vi "Motor_Control.vi"() -> ()   [LabVIEW 2024]
panel:
  out "MotorPosition":i32
  in  "B1":bool
  in  "B10000":bool
  in  "B50000":bool
  in  "B200000":bool
  in  "F200000":bool
  in  "F50000":bool
  in  "F10000":bool
  in  "F1":bool
  in  "Stop":bool
  out "ZMotorTrace":dbl(graph)
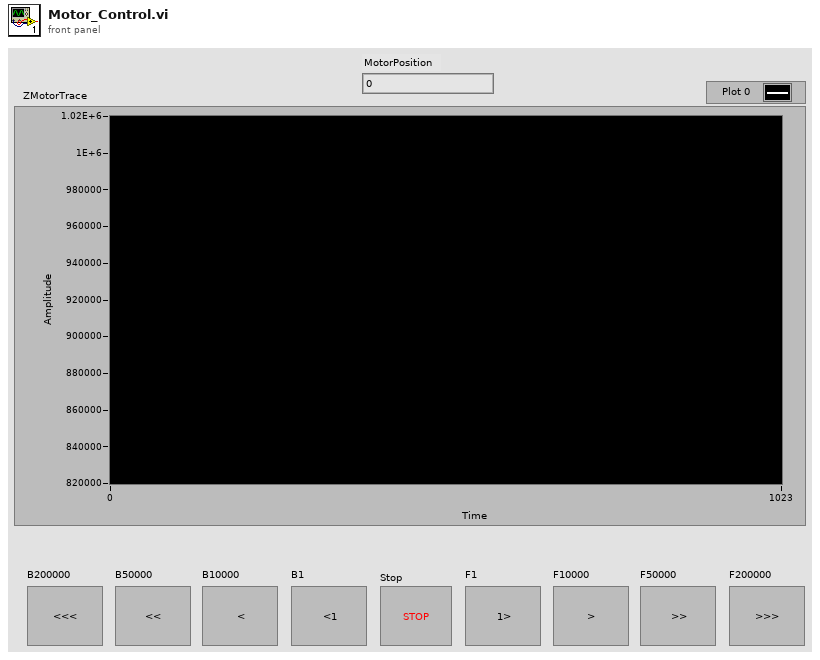
[diagram p1: front panel]
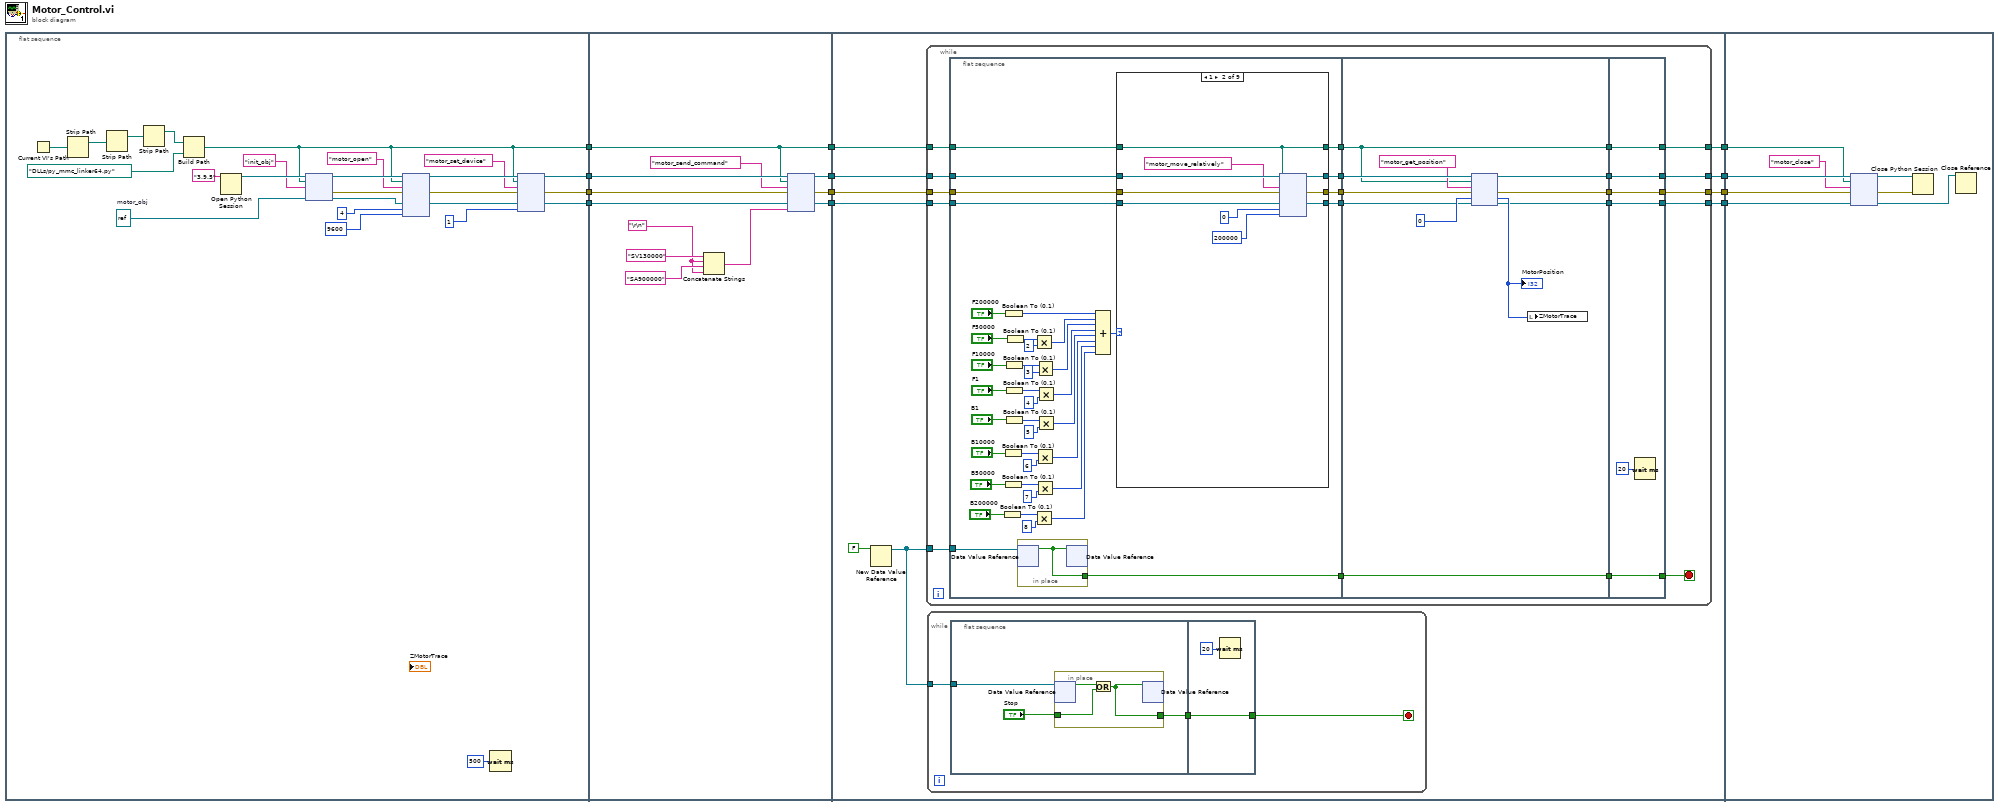
[diagram p0: block diagram]
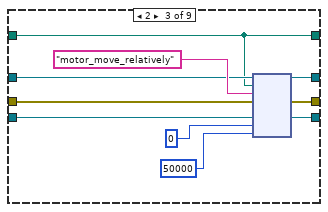
[diagram p3: hidden frame]
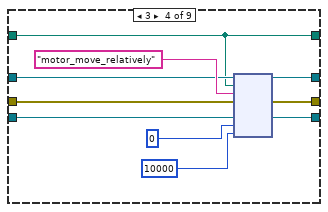
[diagram p4: hidden frame]
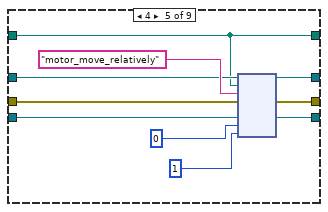
[diagram p5: hidden frame]
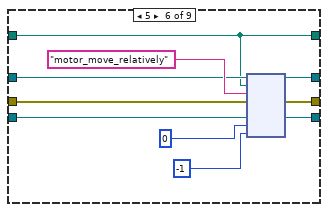
[diagram p6: hidden frame]
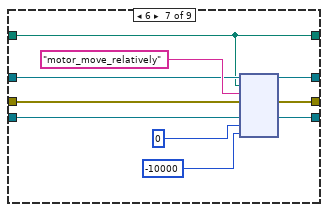
[diagram p7: hidden frame]
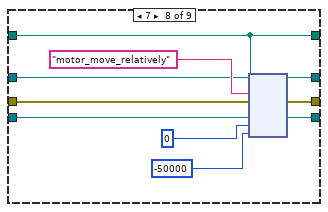
[diagram p8: hidden frame]
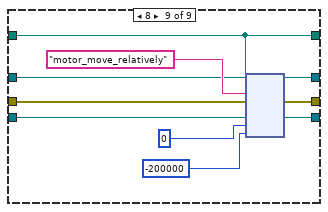
[diagram p9: hidden frame]
diagram:
  n1 = flat-sequence {
    tunnel: [w13] -> w12
    tunnel: [w19] -> w11
    tunnel: [w18] -> w10
    tunnel: [w17] -> w9
    tunnel: w12 -> [w42]
    tunnel: w11 -> [w47]
    tunnel: w10 -> [w46]
    tunnel: w9 -> [w45]
    tunnel: [w42] -> w8
    tunnel: [w41] -> w7
    tunnel: [w40] -> w6
    tunnel: [w39] -> w5
    tunnel: w8 -> [w57]
    tunnel: w7 -> [w56]
    tunnel: w6 -> [w55]
    tunnel: w5 -> [w54]
    tunnel: [w53] -> w4
    tunnel: [w52] -> w3
    tunnel: [w51] -> w2
    tunnel: [w50] -> w1
    tunnel: w4 -> [w238]
    tunnel: w3 -> [w241]
    tunnel: w2 -> [w239]
    tunnel: w1 -> [w240]
    frame #0 {
      w30 = refnum<k38> refnum  # motor_obj
      n2 = Current VI's Path() -> (path=w34:path)
      n3 = Strip Path(path=w34) -> (stripped path=w33:path)  [unwired: 1 out]
      n4 = Strip Path(path=w33) -> (stripped path=w15:path)  [unwired: 1 out]
      n5 = Strip Path(path=w15) -> (stripped path=w14:path)  [unwired: 1 out]
      n6 = Build Path(base path=w14, name or relative path=path "DLLs/py_mmc_linker64.py") -> (appended path=w13:path)
      n7 = Open Python Session(python version="3.9.5" ("Python version")) -> (session out=w35:refnum<k35>)  [unwired: 2 in, 1 out]
      n8 = node(w35, w13, "init_obj" ("function name"), w30) -> (w29:refnum<k35>, w28:errorcluster, w26:refnum<k38>)  [unwired: 1 in, 2 out]
      n9 = node(w29, w13, "motor_open" ("function name"), w28, w26, u8 4 ("COM port select"), 9600 ("COM port select")) -> (w23:refnum<k35>, w22:errorcluster, w21:refnum<k38>)  [unwired: 4 in, 2 out]
      n10 = Wait (ms)(milliseconds to wait=u32 500) -> ()  [unwired: 1 out]
      n11 = node(w23, w13, "motor_set_device" ("function name"), w22, w21, u8 1 ("COM port select")) -> (w19:refnum<k35>, w18:errorcluster, w17:refnum<k38>)  [unwired: 3 in, 2 out]
    }
    frame #1 {
      w38 = "\r\n"
      n12 = Concatenate Strings("SV130000", w38, "SA900000", w38) -> (w44:string)
      n13 = node(w47, w42, "motor_send_command" ("function name"), w46, w45, w44) -> (w41:refnum<k35>, w40:errorcluster, w39:refnum<k38>)  [unwired: 3 in, 2 out]
    }
    frame #2 {
      n14 = New Data Value Reference(data value=FALSE) -> (data value reference=w58:refnum<data-value>)  [unwired: 1 in, 1 out]
      n15 = while {
        tunnel: w58 -> [w90]
        tunnel: w57 -> [w86]
        tunnel: w56 -> [w85]
        tunnel: w55 -> [w84]
        tunnel: w54 -> [w83]
        tunnel: [w77] -> w53
        tunnel: [w75] -> w52
        tunnel: [w73] -> w51
        tunnel: [w71] -> w50
        stop <- w89 stop-if-true
        n16 = flat-sequence {
          tunnel: w90 -> [w131]
          tunnel: [w130] -> w88
          tunnel: w86 -> [w98]
          tunnel: w85 -> [w97]
          tunnel: w84 -> [w96]
          tunnel: w83 -> [w95]
          tunnel: [w94] -> w82
          tunnel: [w93] -> w81
          tunnel: [w92] -> w80
          tunnel: [w91] -> w79
          tunnel: w88 -> [w227]
          tunnel: [w227] -> w87
          tunnel: w82 -> [w226]
          tunnel: w81 -> [w225]
          tunnel: w80 -> [w219]
          tunnel: w79 -> [w221]
          tunnel: [w221] -> w78
          tunnel: [w220] -> w76
          tunnel: [w218] -> w74
          tunnel: [w217] -> w72
          tunnel: [w233] -> w89
          tunnel: w87 -> [w233]
          tunnel: w78 -> [w231]
          tunnel: [w231] -> w77
          tunnel: w76 -> [w230]
          tunnel: [w230] -> w75
          tunnel: [w229] -> w73
          tunnel: w74 -> [w229]
          tunnel: w72 -> [w228]
          tunnel: [w228] -> w71
          frame #0 {
            n17 = Boolean To (0,1)(Boolean="B200000") -> (0, 1=w102:i16)
            n18 = Boolean To (0,1)(Boolean="B10000") -> (0, 1=w110:i16)
            n19 = Boolean To (0,1)(Boolean="B50000") -> (0, 1=w105:i16)
            n20 = Boolean To (0,1)(Boolean="F200000") -> (0, 1=w128:i16)
            n21 = Boolean To (0,1)(Boolean="F10000") -> (0, 1=w121:i16)
            n22 = Boolean To (0,1)(Boolean="F1") -> (0, 1=w117:i16)
            n23 = Boolean To (0,1)(Boolean="B1") -> (0, 1=w113:i16)
            n24 = Boolean To (0,1)(Boolean="F50000") -> (0, 1=w125:i16)
            n25 = in-place {
              in-place-border: [w216] -> w130
              n26 = in-place-dvr #1(w131) -> (w216:bool)  [unwired: 1 out]
              n27 = in-place-dvr #1(w216) -> ()  [unwired: 2 out]
            }
            n28 = Multiply(x=w125, y=i16 2) -> (x*y=w123:i16)
            n29 = Multiply(x=w102, y=i16 8) -> (x*y=w99:i16)
            n30 = Multiply(x=w110, y=i16 6) -> (x*y=w107:i16)
            n31 = Multiply(x=w105, y=i16 7) -> (x*y=w103:i16)
            n32 = Multiply(x=w121, y=i16 3) -> (x*y=w119:i16)
            n33 = Multiply(x=w117, y=i16 4) -> (x*y=w115:i16)
            n34 = Multiply(x=w113, y=i16 5) -> (x*y=w111:i16)
            n35 = Compound Arithmetic op=ADD(w128, w123, w119, w115, w111, w107, w103, w99) -> (w127:i16)
            n36 = case shown="1" w127 {
              tunnel: w98 -> [w135 w136 w151 w156 w166 w176 w186 w196 w206]
              tunnel: w97 -> [w134 w145 w152 w162 w172 w182 w192 w202 w212]
              tunnel: w96 -> [w133 w144 w149 w161 w170 w180 w190 w200 w210]
              tunnel: w95 -> [w132 w143 w147 w160 w168 w178 w188 w198 w208]
              tunnel: [w134 w139 w150 w159 w171 w181 w191 w201 w211] -> w94
              tunnel: [w133 w138 w148 w158 w169 w179 w189 w199 w209] -> w93
              tunnel: [w132 w137 w146 w157 w167 w177 w187 w197 w207] -> w92
              tunnel: [w135 w136 w151 w156 w166 w176 w186 w196 w206] -> w91
              frame 0, Default {
              }
              frame 1 {
                n37 = node(w145, w136, "motor_move_relatively" ("function name"), w144, w143, 0 ("Axis (0..16)"), 200000 ("Position Shift [counts]")) -> (w139:refnum<k35>, w138:errorcluster, w137:refnum<k38>)  [unwired: 4 in, 2 out]
              }
              frame 2 {
                n38 = node(w152, w151, "motor_move_relatively" ("function name"), w149, w147, 0 ("Axis (0..16)"), 50000 ("Position Shift [counts]")) -> (w150:refnum<k35>, w148:errorcluster, w146:refnum<k38>)  [unwired: 4 in, 2 out]
              }
              frame 3 {
                n39 = node(w162, w156, "motor_move_relatively" ("function name"), w161, w160, 0 ("Axis (0..16)"), 10000 ("Position Shift [counts]")) -> (w159:refnum<k35>, w158:errorcluster, w157:refnum<k38>)  [unwired: 4 in, 2 out]
              }
              frame 4 {
                n40 = node(w172, w166, "motor_move_relatively" ("function name"), w170, w168, 0 ("Axis (0..16)"), 1 ("Position Shift [counts]")) -> (w171:refnum<k35>, w169:errorcluster, w167:refnum<k38>)  [unwired: 4 in, 2 out]
              }
              frame 5 {
                n41 = node(w182, w176, "motor_move_relatively" ("function name"), w180, w178, 0 ("Axis (0..16)"), -1 ("Position Shift [counts]")) -> (w181:refnum<k35>, w179:errorcluster, w177:refnum<k38>)  [unwired: 4 in, 2 out]
              }
              frame 6 {
                n42 = node(w192, w186, "motor_move_relatively" ("function name"), w190, w188, 0 ("Axis (0..16)"), -10000 ("Position Shift [counts]")) -> (w191:refnum<k35>, w189:errorcluster, w187:refnum<k38>)  [unwired: 4 in, 2 out]
              }
              frame 7 {
                n43 = node(w202, w196, "motor_move_relatively" ("function name"), w200, w198, 0 ("Axis (0..16)"), -50000 ("Position Shift [counts]")) -> (w201:refnum<k35>, w199:errorcluster, w197:refnum<k38>)  [unwired: 4 in, 2 out]
              }
              frame 8 {
                n44 = node(w212, w206, "motor_move_relatively" ("function name"), w210, w208, 0 ("Axis (0..16)"), -200000 ("Position Shift [counts]")) -> (w211:refnum<k35>, w209:errorcluster, w207:refnum<k38>)  [unwired: 4 in, 2 out]
              }
            }
          }
          frame #1 {
            n45 = node(w226, w221, "motor_get_position" ("function name"), w225, 0, w219) -> (w220:refnum<k35>, w217:errorcluster, w222:i32, w218:refnum<k38>)  [unwired: 2 out]
            "MotorPosition" <- w222
            n46 = local write "ZMotorTrace"(w222) -> ()
          }
          frame #2 {
            n47 = Wait (ms)(milliseconds to wait=u32 20) -> ()  [unwired: 1 out]
          }
        }
      }
      n48 = while {
        tunnel: w58 -> [w62]
        stop <- w60 stop-if-true
        n49 = flat-sequence {
          tunnel: w62 -> [w65]
          tunnel: [w63] -> w61
          tunnel: [w69] -> w60
          tunnel: w61 -> [w69]
          frame #0 {
            n50 = in-place {
              in-place-border: "Stop" -> [w67]
              in-place-border: [w66] -> w63
              n51 = in-place-dvr #2(w65) -> (w68:bool)  [unwired: 1 out]
              n52 = Or(x=w68, y=w67) -> (x .or. y?=w66:bool)
              n53 = in-place-dvr #2(w66) -> ()  [unwired: 2 out]
            }
          }
          frame #1 {
            n54 = Wait (ms)(milliseconds to wait=u32 20) -> ()  [unwired: 1 out]
          }
        }
      }
    }
    frame #3 {
      n55 = node(w241, w238, "motor_close" ("function name"), w240, w239) -> (w236:refnum<k35>, w235:errorcluster, w234:refnum<k38>)  [unwired: 2 in, 2 out]
      n56 = Close Python Session(session in=w236, error in=w235) -> ()  [unwired: 1 out]
      n57 = Close Reference(reference=w234) -> ()  [unwired: 1 in, 1 out]
    }
  }
